vi "3D-AutoCreatListName.vi"() -> (1 "ListRowName":string[](array[string]), 2 "ListColName":string[](array[string]), 3 "ListValueName":string[][](array[string]))   [LabVIEW 2015]
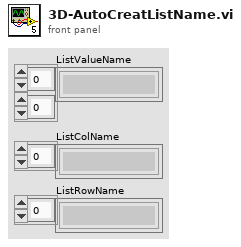
[diagram p1: front panel]
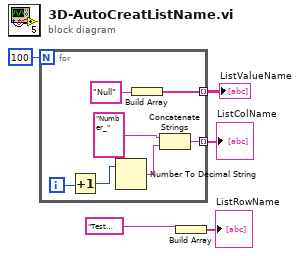
[diagram p0: block diagram]
diagram:
  n1 = for {
    N: 100 -> [_]
    tunnel: [w11] -> w3 mode=indexing
    tunnel: [w6] -> w2 mode=indexing
    i -> [w10]
    n2 = Increment(x=w10) -> (x+1=w9:i32)
    n3 = Number To Decimal String(number=w9) -> (decimal integer string=w7:string)  [unwired: 1 in]
    n4 = Build Array("Null") -> (w11:string[])
    n5 = Concatenate Strings("Number_", w7) -> (w6:string)
  }
  "ListValueName" <- w3
  "ListColName" <- w2
  n6 = Build Array("Test Value") -> (→"ListRowName":string[])
